vi "Constructor.vi"(8 "error in (no error)":errorcluster, 10 "FPGA Target Name":string, 11 "Project Path":path) -> (0 "error out":errorcluster, 3 "Project out":refnum<class "Project.lvclass">)   [LabVIEW 2025, in "Project.lvclass"]
doc: "Open LV Project Ref and replace autogenerated folder for dynamically added items (DMA, memory, etc)."
uses:
  Project.lvclass
  Project.lvclass/Project.ctl
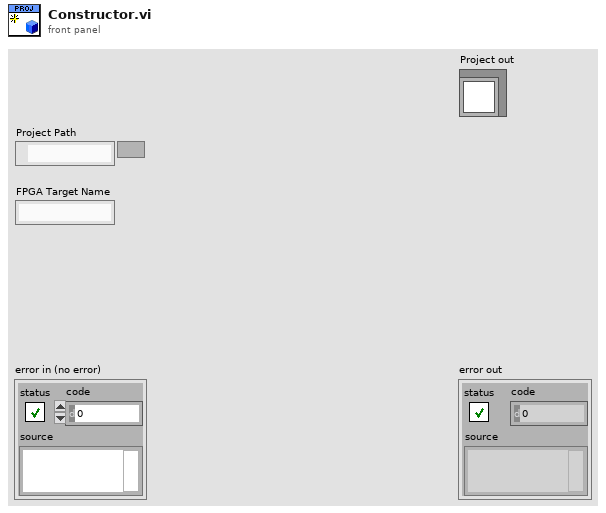
[diagram p1: front panel]
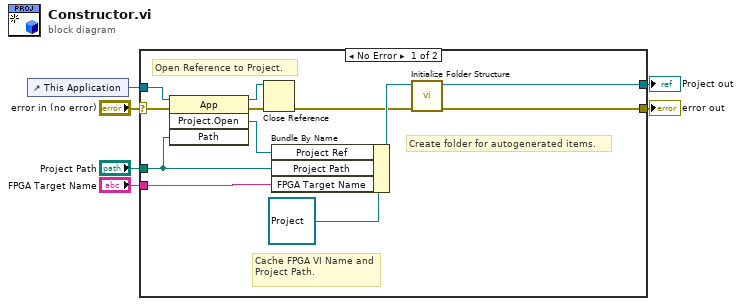
[diagram p0: block diagram]
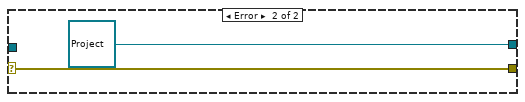
[diagram p2: hidden frame]
diagram:
  n1 = control-ref of="This Application"() -> (w1:refnum<vi>)
  n2 = case shown="No Error" "error in (no error)" {
    selector: "error in (no error)" -> [w15 w20]
    tunnel: [w14 w20] -> w5
    tunnel: [w12 refnum<class "Project.lvclass"> refnum ("Project out")] -> w4
    tunnel: "Project Path" -> [w10 _]
    tunnel: "FPGA Target Name" -> [w9 _]
    tunnel: w1 -> [w8 _]
    frame No Error {
      # "Open Reference to Project."
      # "Create folder for autogenerated items."
      # "Cache FPGA VI Name and Project Path."
      n3 = invoke class="App" method="Project.Open"(reference=w8, error in=w15, "Path"=w10) -> (reference out=w17:refnum<vi>, error out=w18:errorcluster, "Project:Open"=w16:refnum<vi>)  [unwired: 1 in, 1 out]
      n4 = Close Reference(reference=w17, error in (no error)=w18) -> (error out=w7:errorcluster)
      n5 = Bundle By Name(cluster=refnum<class "Project.lvclass"> refnum ("Project out"), "Project Ref"=w16, "Project Path"=w10, "FPGA Target Name"=w9) -> (w13:refnum<class "Project.lvclass">)
      n6 = call-dynamic "Initialize Folder Structure.vi"("error in (no error)"=w7, "Project in"=w13) -> ("error out"=w14:errorcluster, "Project out"=w12:refnum<class "Project.lvclass">)  [unwired: 8 in]
    }
    frame Error {
    }
  }
  "error out" <- w5
  "Project out" <- w4
